vi "SetArmDirection.vi"(8 "Error In":errorcluster, 10 "Arm Direction":T1, 11 "Keithley 6482 In":refnum<visa-resource-name>) -> (0 "Error Out":errorcluster, 3 "Keithley 6482 Out":refnum<visa-resource-name>)   [LabVIEW 2009, in "Keithley-6482-Visa.lvlib"]
uses:
  <instrlib>/Keithley-6482-Visa9.0/Keithley-6482-Visa.lvlib
  <instrlib>/Keithley-6482-Visa9.0/Public/Controls/ArmDirection.ctl
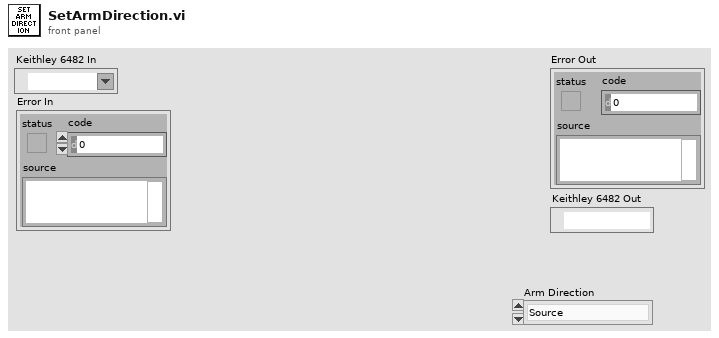
[diagram p1: front panel]
types:
  T1 = typedef "Keithley-6482-Visa.lvlib/ArmDirection.ctl" = enum16{"Source", "Acceptor"}
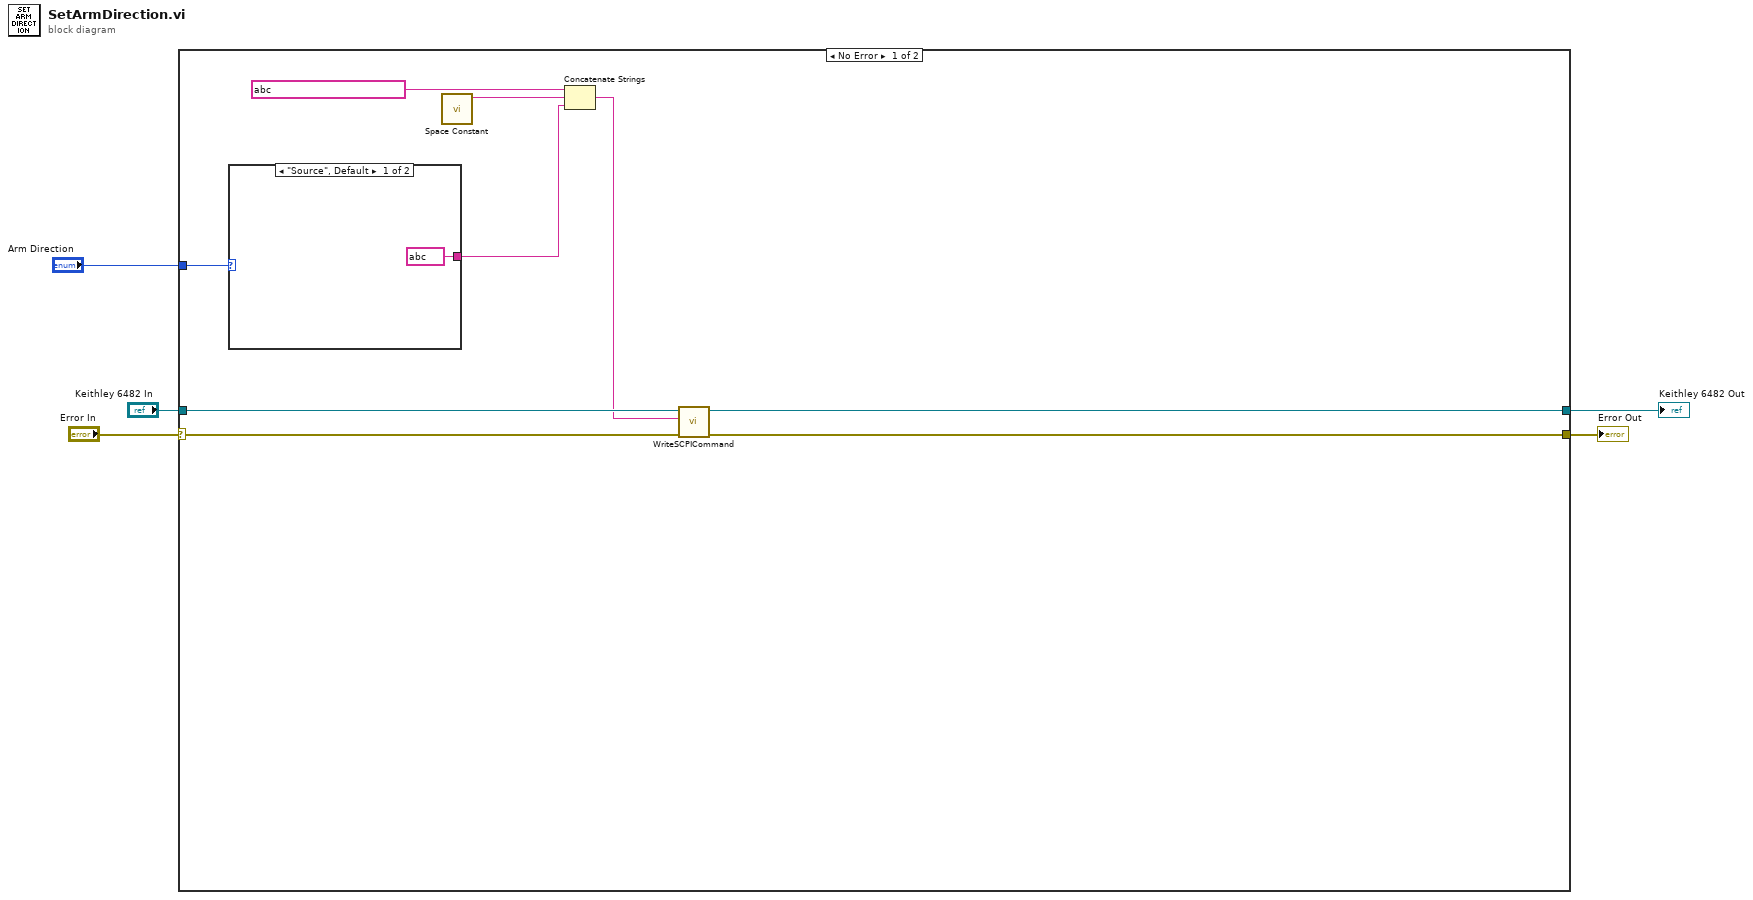
[diagram p0: block diagram]
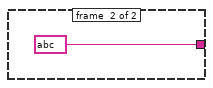
[diagram p2: hidden frame]
diagram:
  n1 = case shown="No Error" "Error In" {
    selector: "Error In" -> [w14 w17]
    tunnel: "Keithley 6482 In" -> [w13 w18]
    tunnel: [w8 w17] -> w3
    tunnel: [w9 w18] -> w2
    tunnel: "Arm Direction" -> [w7 _]
    frame #0 {
      n2 = case shown="\"Source\", Default" w7 {
        tunnel: [string ? string ?] -> w6
        frame #0 {
        }
        frame #1 {
        }
      }
      n3 = call <vilib>:"Space Constant.vi"() -> ("String"=w11:string)
      n4 = Concatenate Strings(string ? ("string"), w11, w6) -> (w10:string)
      n5 = call <instrlib>:"WriteSCPICommand.vi"("Error In"=w14, "SCPI Command"=w10, "Keithley 6482 In"=w13) -> ("Error Out"=w8:errorcluster, "Keithley 6482 Out"=w9:refnum<visa-resource-name>)  [unwired: 7 in]
    }
    frame #1 {
    }
  }
  "Error Out" <- w3
  "Keithley 6482 Out" <- w2
